vi "Get Channel Information.vi"(8 "error in (no error)":errorcluster, 11 "Potentiostat Galvanostat in":refnum<class "Potentiostat Galvanostat.lvclass">) -> (0 "error out":errorcluster, 2 "Channel Information":T1 {"Channel" items=["Channel 0", "Channel 1", "Channel 2", "Channel 3", "Channel 4", "Channel 5", "Channel 6", "Channel 7", "Channel 8", "Channel 9", "Channel 10", "Channel 11", "Channel 12", "Channel 13", "Channel 14", "Channel 15"]; "Firmware Code" items=["No firmware loaded"=0, "Firmware for EC-Lab software"=1, "Unknown firmware loaded"=4, "Firmware for the library"=5, "Invalid firmware loaded"=8, "Firmware for calibration software"=10]; "Amplifier Code" items=["No amplifier VMP3 series"=0, "Amplifier 2 A VMP3 series"=1, "Amplifier 1 A VMP3 series"=2, "Amplifier 5 A VMP3 series"=3, "Amplifier 10 A VMP3 series"=4, "Amplifier 20 A VMP3 series"=5, "reserved VMP3 series"=6, "Low current amplifier VMP3 series"=7, "Amplifier 80 A VMP3 series"=8, "Amplifier 4 A VMP3 series"=9, "Fuel Cell Tester VMP3 series"=10, "Amplifier 4 A (VSP instrument) VMP3 series"=11, "Low current amplifier (VSP instrument) VMP3 series"=12, "Undefined amplifier VMP3 series"=13, "reserved VMP3 series"=14, "No amplifier VMP3 series"=15, "Amplifier 8 A VMP3 series"=16, "Amplifier LB500 VMP3 series"=17, "Amplifier 100 A VMP3 series"=18, "Amplifier LB2000 VMP3 series"=19, "Amplifier 1A 48V SP-300 series"=20, "Amplifier 4A 14V SP-300 series"=21, "MPG-205 5A amplifier"=22, "MPG-210 10A amplifier"=23, "MPG-220 20A amplifier"=24, "MPG-240 40A amplifier"=25, "coin cell holder"=26, "VMP4 10A/5V amplifier (SP-300 internal amplifier)"=27, "VMP4 2A/30V"=28, "VMP4 1A/48VP"=129]; "Channel State" items=["Channel is stopped", "Channel is running", "Channel is paused"]; "Maximum Current Range Allowed" items=["I range 100 pA SP-300 series", "I range 1 nA VMP3 / SP-300 series", "I range 10 nA VMP3 / SP-300 series", "I range 100 nA VMP3 / SP-300 series", "I range 1 uA VMP3 / SP-300 series", "I range 10 uA VMP3 / SP-300 series", "I range 100 uA VMP3 / SP-300 series", "I range 1 mA VMP3 / SP-300 series", "I range 10 mA VMP3 / SP-300 series", "I range 100 mA VMP3 / SP-300 series", "I range 1 A VMP3 / SP-300 series", "Booster VMP3 / SP-300 series", "Auto range VMP3 / SP-300 series"]; "Minimum Current Range Allowed" items=["I range 100 pA SP-300 series", "I range 1 nA VMP3 / SP-300 series", "I range 10 nA VMP3 / SP-300 series", "I range 100 nA VMP3 / SP-300 series", "I range 1 uA VMP3 / SP-300 series", "I range 10 uA VMP3 / SP-300 series", "I range 100 uA VMP3 / SP-300 series", "I range 1 mA VMP3 / SP-300 series", "I range 10 mA VMP3 / SP-300 series", "I range 100 mA VMP3 / SP-300 series", "I range 1 A VMP3 / SP-300 series", "Booster VMP3 / SP-300 series", "Auto range VMP3 / SP-300 series"]; "Maximum Bandwidth" items=["Bandwidth #1"=1, "Bandwidth #2"=2, "Bandwidth #3"=3, "Bandwidth #4"=4, "Bandwidth #5"=5, "Bandwidth #6"=6, "Bandwidth #7"=7, "Bandwidth #8 (only with SP-300 series)"=8, "Bandwidth #9 (only with SP-300 series)"=9]}, 3 "Potentiostat Galvanostat out":refnum<class "Potentiostat Galvanostat.lvclass">)   [LabVIEW 2018, in "Potentiostat Galvanostat.lvclass"]
uses:
  Potentiostat Galvanostat.lvclass
  Controls/Channel Information.ctl
  Controls/Channel.ctl
  Controls/Firmware Code.ctl
  Controls/Amplifier Type.ctl
  Controls/Channel State.ctl
  Controls/Current Range.ctl
  Controls/Bandwidth.ctl
  Potentiostat Galvanostat.lvclass/Potentiostat Galvanostat.ctl
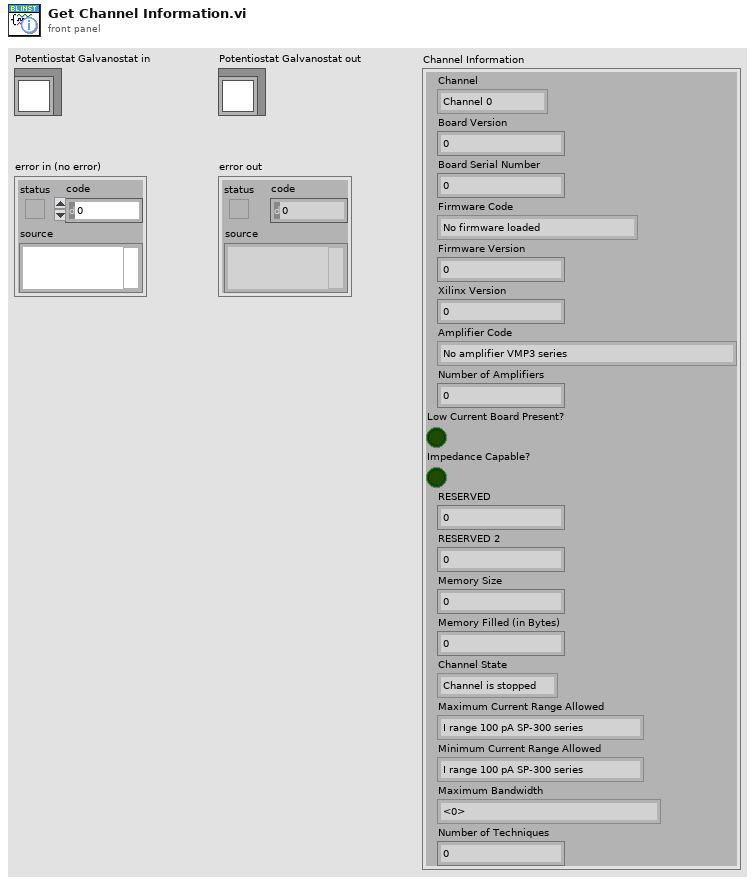
[diagram p1: front panel]
types:
  T1 = typedef "Potentiostat Galvanostat.lvclass/Channel Information.ctl" = cluster{"Channel":T2, "Board Version":i32, "Board Serial Number":i32, "Firmware Code":T3, "Firmware Version":i32, "Xilinx Version":i32, "Amplifier Code":T4, "Number of Amplifiers":i32, "Low Current Board Present?":bool, "Impedance Capable?":bool, "RESERVED":i32, "RESERVED 2":i32, "Memory Size":i32, "Memory Filled (in Bytes)":i32, "Channel State":T5, "Maximum Current Range Allowed":T6, "Minimum Current Range Allowed":T6, "Maximum Bandwidth":T7, "Number of Techniques":i32}
  T2 = typedef "Potentiostat Galvanostat.lvclass/Channel.ctl" = u8
  T3 = typedef "Potentiostat Galvanostat.lvclass/Firmware Code.ctl" = i32
  T4 = typedef "Potentiostat Galvanostat.lvclass/Amplifier Type.ctl" = i32
  T5 = typedef "Potentiostat Galvanostat.lvclass/Channel State.ctl" = i32
  T6 = typedef "Potentiostat Galvanostat.lvclass/Current Range.ctl" = i32
  T7 = typedef "Potentiostat Galvanostat.lvclass/Bandwidth.ctl" = i32
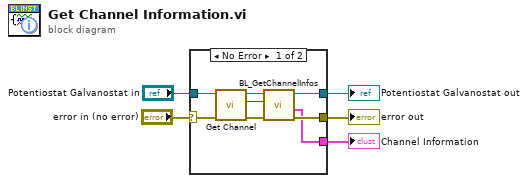
[diagram p0: block diagram]
diagram:
  n1 = case shown="No Error" "error in (no error)" {
    selector: "error in (no error)" -> [w12 w15]
    tunnel: [w7 w15] -> w4
    tunnel: [w9 w14] -> w2
    tunnel: "Potentiostat Galvanostat in" -> [w13 w14]
    tunnel: [w6 _] -> w1
    frame No Error {
      n2 = call "Get Channel.vi"("error in (no error)"=w12, "Potentiostat Galvanostat in"=w13) -> ("error out"=w10:errorcluster, "Channel"=w8:T2, "Potentiostat Galvanostat out"=w11:refnum<class "Potentiostat Galvanostat.lvclass">)  [unwired: 7 in]
      n3 = call "BL_GetChannelInfos.vi"("error in (no error)"=w10, "Channel"=w8, "Potentiostat Galvanostat in"=w11) -> ("error out"=w7:errorcluster, "Channel Information"=w6:T1, "Potentiostat Galvanostat out"=w9:refnum<class "Potentiostat Galvanostat.lvclass">)  [unwired: 5 in, 1 out]
    }
    frame Error {
    }
  }
  "error out" <- w4
  "Potentiostat Galvanostat out" <- w2
  "Channel Information" <- w1
